vi "Read Byte Count.vi"(8 "error in (no error)":errorcluster, 11 "ReadCommand in":refnum<class "ReadCommand.lvclass">) -> (0 "error out":errorcluster, 2 "Byte Count":u32 step=1 format="%.0g", 3 "ReadCommand out":refnum<class "ReadCommand.lvclass">)   [LabVIEW 2023, in "HAF.lvlib" / "ReadCommand.lvclass"]
doc: "Returns the current Byte Count. If zero, then 1024 is returned."
uses:
  ReadCommand.lvclass
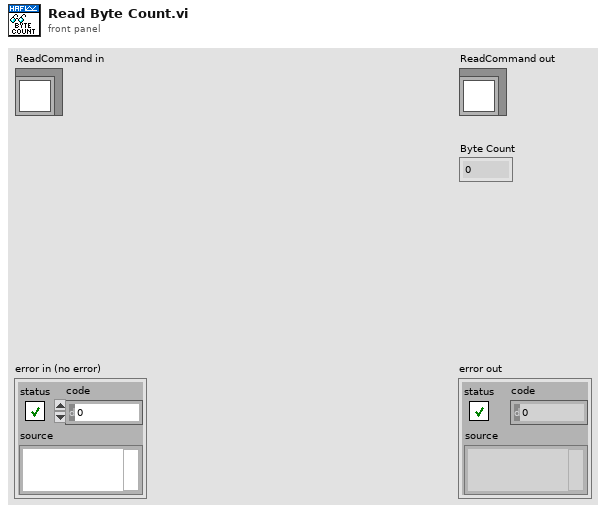
[diagram p1: front panel]
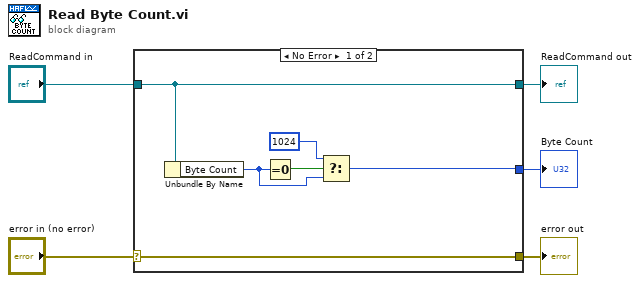
[diagram p0: block diagram]
diagram:
  n1 = case shown="No Error" "error in (no error)" {
    selector: "error in (no error)" -> [w11 w12]
    tunnel: [w11 w12] -> w4
    tunnel: [w10 w13] -> w2
    tunnel: "ReadCommand in" -> [w10 w13]
    tunnel: [w6 _] -> w1
    frame No Error {
      n2 = Unbundle By Name(w10) -> ("Byte Count"=w7:u32)
      n3 = Equal To 0?(x=w7) -> (x = 0?=w9:bool)
      n4 = Select(t=u32 1024, s=w9, f=w7) -> (s? t:f=w6:u32)
    }
    frame Error {
    }
  }
  "error out" <- w4
  "ReadCommand out" <- w2
  "Byte Count" <- w1
